vi "HEWH Agilent Add Calibration Data.vi"(8 "Error In":errorcluster, 9 "Sorted Agilent Data":dbl[](array[numeric]), 11 "Agilent Cluster Array":T1[](array[typedef])) -> (0 "Error Out":errorcluster, 2 "Agilent Raw Cluster Array":T1[](array[typedef]), 3 "Agilent Calibrated Cluster Array":T1[](array[typedef]))   [LabVIEW 2016]
uses:
  Type Definitions/HEWH Agilent Cluster.ctl
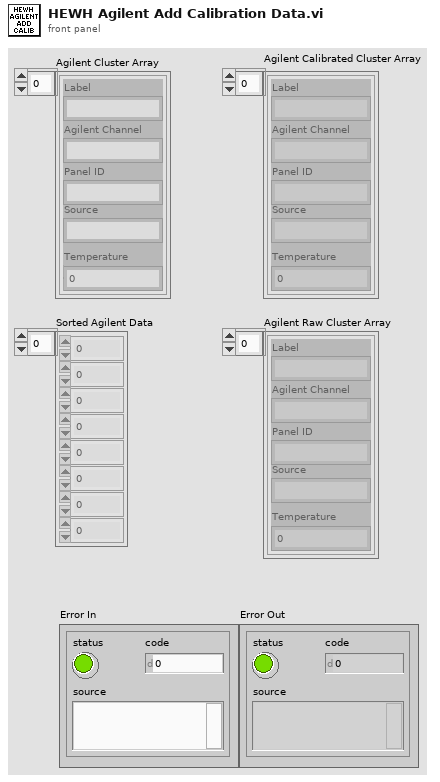
[diagram p1: front panel]
types:
  T1 = typedef "HEWH Agilent Cluster.ctl" = cluster{"Label":string, "Agilent Channel":string, "Panel ID":string, "Source":string, "Temperature":dbl}
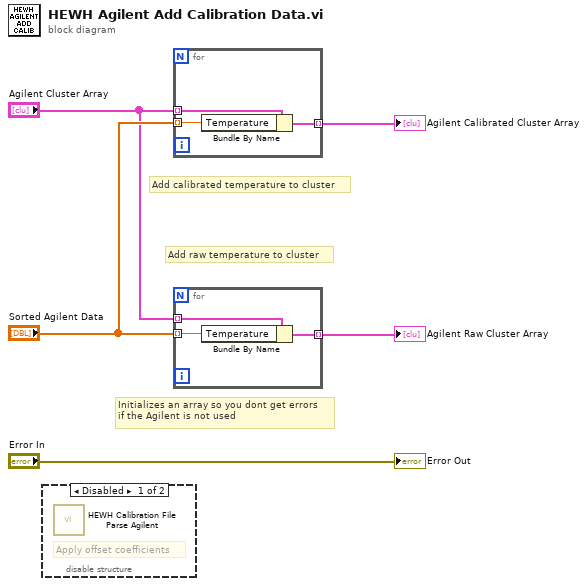
[diagram p0: block diagram]
diagram:
  # "Add calibrated temperature to cluster"
  # "Add raw temperature to cluster"
  # "Initializes an array so you dont get errors \nif the Agilent is not used"
  n1 = disable-structure shown="Disabled" {
    frame Disabled {
      # "Apply offset coefficients"
      n2 = call "HEWH Calibration File Parse Agilent.vi"() -> ()  [unwired: 8 in, 2 out]
    }
    frame Enabled {
    }
  }
  n3 = for {
    tunnel: "Agilent Cluster Array" -> [w8] mode=indexing
    tunnel: "Sorted Agilent Data" -> [w7] mode=indexing
    tunnel: [w6] -> w3 mode=indexing
    n4 = Bundle By Name(cluster=w8, "Temperature"=w7) -> (w6:T1)
  }
  "Agilent Calibrated Cluster Array" <- w3
  n5 = for {
    tunnel: "Agilent Cluster Array" -> [w11] mode=indexing
    tunnel: "Sorted Agilent Data" -> [w10] mode=indexing
    tunnel: [w9] -> w2 mode=indexing
    n6 = Bundle By Name(cluster=w11, "Temperature"=w10) -> (w9:T1)
  }
  "Agilent Raw Cluster Array" <- w2
  "Error Out" <- "Error In"
